vi "GetShapeResultNames.vi"(7 "ProjectName":string="Prj", 10 "SetParameter":T1={"Enum_ShapeType"=enum."Circles", "MaxParticle"=1, "Descriptor"={"Set 1"=100.0, "Set 2"=10.0, "Set 3"=200.0, "Set 4"=10.0}, "Match Options"={"Rotation"=TRUE, "Scale"=FALSE, "Occlusion"=FALSE, "Range Settings"=[{"Match Constraints"=0, "Min"=0.0, "Max"=360.0}]}, "Curve Parameters"={"Extraction Mode"=0, "Edge Threshold"=75, "Edge Filter Size"=1, "Min Length"=25, "Row Search Step Size"=15, "Col Search Step Size"=15, "Max Endpoint Gap"=10, "Closed"=FALSE, "Subpixel"=FALSE}, " score"=500.0} {"score" format="%#_15g"; "Curve Parameters"."Extraction Mode" items=["Normal", "Uniform Regions"]; "Curve Parameters"."Edge Filter Size" items=["Fine", "Normal"]; "Match Options"."Range Settings"."Match Constraints" items=["Rotation Angle (degrees)", "Scale Factor (%)", "Occlusion (%)"]}, 11 "ROI_Name":string="ROI1") -> (3 "ResultNames":string[](array[string]))   [LabVIEW 2019]
uses:
  Controls/Circle/Analysis_Circle_Result.ctl
  Controls/ShapeDectect/Analysis_ShapeDectect_Parameter.ctl
panel:
  in  "Tab Control":T2(tab)
  in  "Circles":T3
  in  "Ellipses":T4
  in  "Lines":T5
  in  "Rectangles":T6
  in  "Analysis_Clamp_Result":T7 {"Fitted Circle"."Average SNR (dB)" format="%.2f"; "Fitted Circle"."Average Strength" format="%.2f"; "Fitted Circle"."Roundness (Real-World)" format="%.2f"; "Fitted Circle"."Radius (Real-World)" format="%.2f"; "Fitted Circle"."Center (Real-World)"."Y" format="%.2f"; "Fitted Circle"."Center (Real-World)"."X" format="%.2f"; "Fitted Circle"."Radius (Pixels)" format="%.2f"; "Fitted Circle"."Center (Pixels)"."Y" format="%.2f"; "Fitted Circle"."Center (Pixels)"."X" format="%.2f"}
  out "error out":errorcluster
  in  "error in (no error)":errorcluster
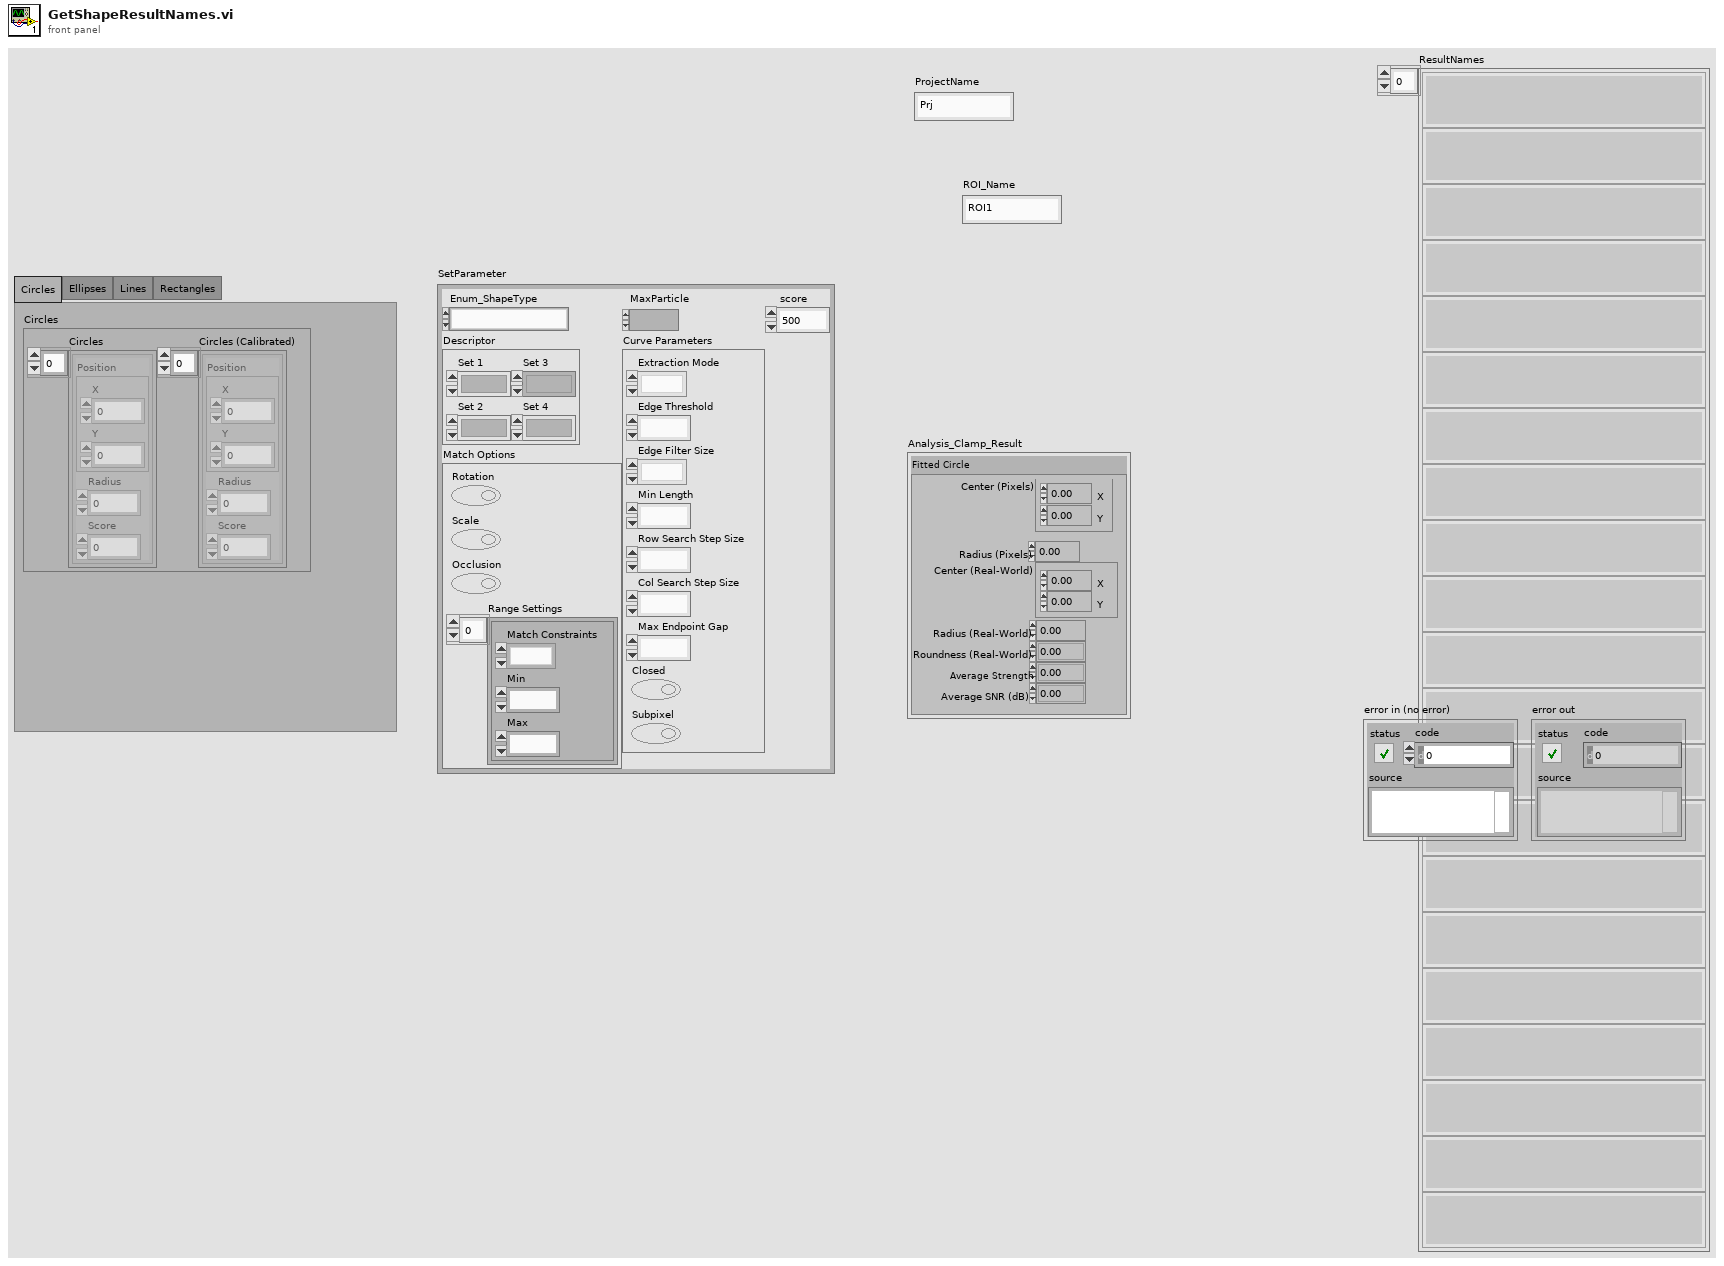
[diagram p1: front panel]
types:
  T1 = typedef "Analysis_ShapeDectect_Parameter.ctl" = cluster{"Enum_ShapeType":enum16{"Circles", "Ellipses", "Lines", "Rectangles"}, "MaxParticle":i32, "Descriptor":cluster{"Set 1":dbl, "Set 2":dbl, "Set 3":dbl, "Set 4":dbl}, "Match Options":cluster{"Rotation":bool, "Scale":bool, "Occlusion":bool, "Range Settings":cluster{"Match Constraints":u32, "Min":dbl, "Max":dbl}[]}, "Curve Parameters":cluster{"Extraction Mode":u32, "Edge Threshold":i32, "Edge Filter Size":u32, "Min Length":i32, "Row Search Step Size":i32, "Col Search Step Size":i32, "Max Endpoint Gap":i32, "Closed":bool, "Subpixel":bool}, " score":dbl}
  T2 = enum32{"Circles", "Ellipses", "Lines", "Rectangles"}
  T3 = cluster{"Circles":cluster{"Position":cluster{"X":sgl, "Y":sgl}, "Radius":dbl, "Score":dbl}[], "Circles (Calibrated)":cluster{"Position":cluster{"X":sgl, "Y":sgl}, "Radius":dbl, "Score":dbl}[]}
  T4 = cluster{"Pixel":cluster{"Position":cluster{"X":sgl, "Y":sgl}, "Angle":dbl, "Major Radius":dbl, "Minor Radius":dbl, "Score":dbl}[], "Ellipses (Calibrated)":cluster{"Position":cluster{"X":sgl, "Y":sgl}, "Orientation":dbl, "Major Radius":dbl, "Minor Radius":dbl, "Score":dbl}[]}
  T5 = cluster{"Lines":cluster{"Start Point":cluster{"X":sgl, "Y":sgl}, "End Point":cluster{"X":sgl, "Y":sgl}, "Length":dbl, "Angle":dbl, "Score":dbl}[], "Lines Calibrated":cluster{"Start Point":cluster{"X":sgl, "Y":sgl}, "End Point":cluster{"X":sgl, "Y":sgl}, "Length":dbl, "Orientation":dbl, "Score":dbl}[]}
  T6 = cluster{"Rectangles":cluster{"Corners":cluster{"X":sgl, "Y":sgl}[], "Angle":dbl, "Width":dbl, "Height":dbl, "Score":dbl}[], "Rectangles Calibrated":cluster{"Corners":cluster{"X":sgl, "Y":sgl}[], "Angle":dbl, "Width":dbl, "Height":dbl, "Score":dbl}[]}
  T7 = typedef "Analysis_Circle_Result.ctl" = cluster{"Fitted Circle":cluster{"Center (Pixels)":cluster{"X":sgl, "Y":sgl}, "Radius (Pixels)":dbl, "Center (Real-World)":cluster{"X":sgl, "Y":sgl}, "Radius (Real-World)":dbl, "Roundness (Real-World)":dbl, "Average Strength":dbl, "Average SNR (dB)":dbl}}
  T8 = enum16{"Circles", "Ellipses", "Lines", "Rectangles"}
  T9 = cluster{"Position":cluster{"X":sgl, "Y":sgl}, "Angle":dbl, "Major Radius":dbl, "Minor Radius":dbl, "Score":dbl}
  T10 = cluster{"Start Point":cluster{"X":sgl, "Y":sgl}, "End Point":cluster{"X":sgl, "Y":sgl}, "Length":dbl, "Angle":dbl, "Score":dbl}
  T11 = cluster{"Corners":cluster{"X":sgl, "Y":sgl}[], "Angle":dbl, "Width":dbl, "Height":dbl, "Score":dbl}
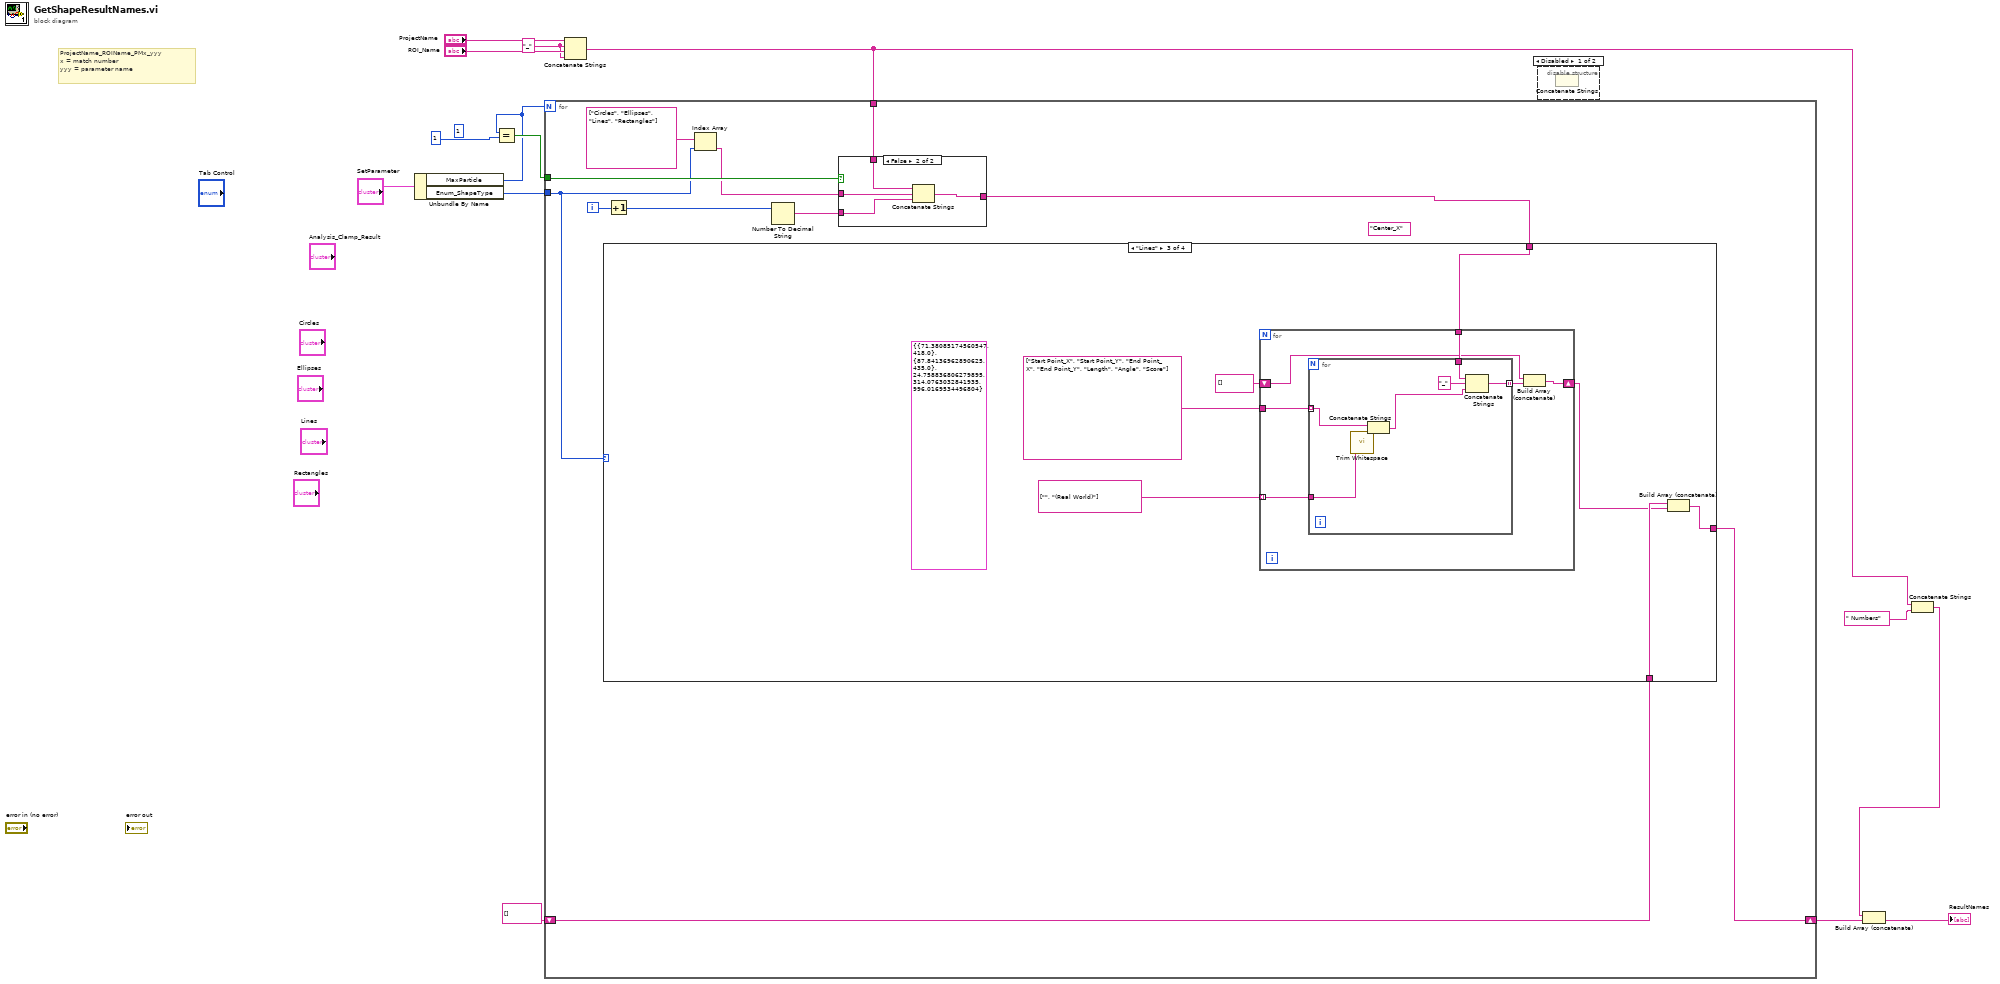
[diagram p0: block diagram]
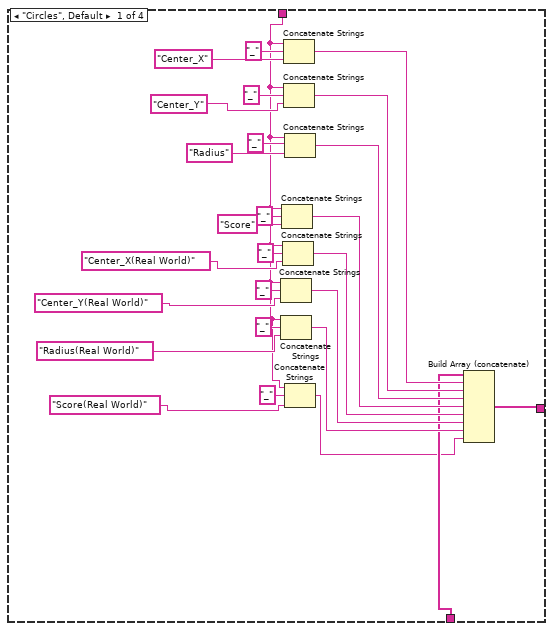
[diagram p3: hidden frame]
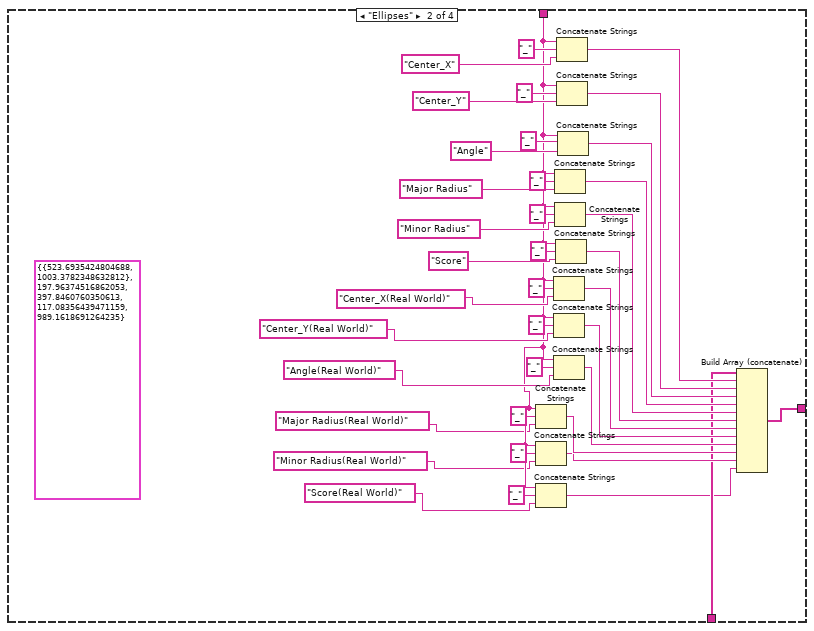
[diagram p4: hidden frame]
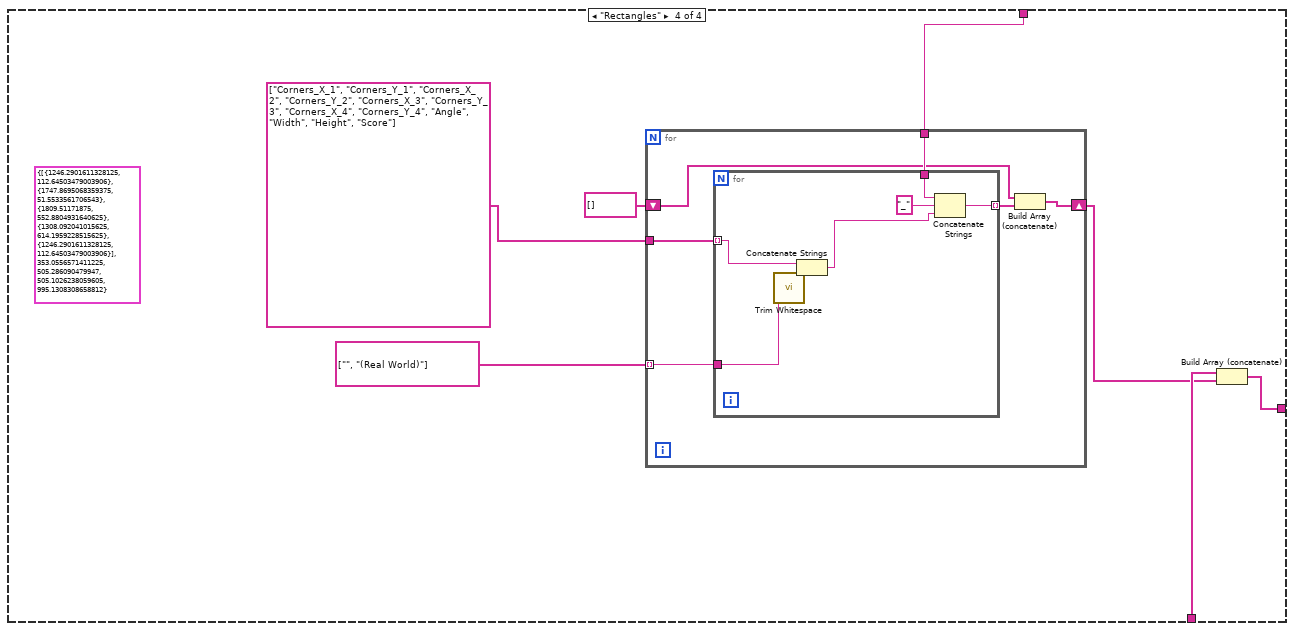
[diagram p5: hidden frame]
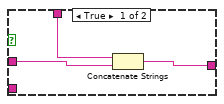
[diagram p6: hidden frame]
diagram:
  (unwired) 1 ("x")
  w12 = "_" ("string")
  # "ProjectName_ROIName_PMx_yyy\nx = match number\nyyy = parameter name"
  n1 = Unbundle By Name("SetParameter") -> ("MaxParticle"=w1:i32, "Enum_ShapeType"=w7:T8)
  n2 = Equal?(x=w1, y=1) -> (x = y?=w9:bool)
  n3 = Concatenate Strings("ProjectName", w12, "ROI_Name", w12) -> (w4:string)
  n4 = for {
    N: w1 -> [_]
    tunnel: w4 -> [w23]
    shift-right: [w19] -> w10
    shift-left: string[] [] -> [w20]
    tunnel: w9 -> [w24]
    tunnel: w7 -> [w15]
    i -> [w21]
    (unwired) "Center_X" ("string")
    n5 = Increment(x=w21) -> (x+1=w25:i32)
    n6 = Index Array(array=string[] ["Circles", "Ellipses", "Lines", "Rectangles"] ("Array"), index=w15) -> (element=w16:string)
    n7 = Number To Decimal String(number=w25) -> (decimal integer string=w22:string)  [unwired: 1 in]
    n8 = case shown="False" w24 {
      tunnel: w23 -> [w134 w138]
      tunnel: w22 -> [_ w136]
      tunnel: [w133 w137] -> w18
      tunnel: w16 -> [w132 w135]
      frame True {
        n9 = Concatenate Strings(w134, w132) -> (w133:string)
      }
      frame False {
        n10 = Concatenate Strings(w138, w135, w136) -> (w137:string)
      }
    }
    n11 = case shown="\"Lines\"" w15 {
      tunnel: w20 -> [w37 w54 w97 w117]
      tunnel: [w38 w91 w98 w118] -> w19
      tunnel: w18 -> [w28 w61 w94 w115]
      frame "Circles", Default {
        n12 = Concatenate Strings(w28, "_" ("string"), "Center_Y(Real World)" ("string")) -> (w48:string)
        n13 = Concatenate Strings(w28, "_" ("string"), "Radius(Real World)" ("string")) -> (w47:string)
        n14 = Concatenate Strings(w28, "_" ("string"), "Score" ("string")) -> (w50:string)
        n15 = Concatenate Strings(w28, "_" ("string"), "Center_X(Real World)" ("string")) -> (w49:string)
        n16 = Concatenate Strings(w28, "_" ("string"), "Center_X" ("string")) -> (w52:string)
        n17 = Concatenate Strings(w28, "_" ("string"), "Center_Y" ("string")) -> (w51:string)
        n18 = Concatenate Strings(w28, "_", "Radius" ("string")) -> (w39:string)
        n19 = Concatenate Strings(w28, "_" ("string"), "Score(Real World)" ("string")) -> (w26:string)
        n20 = Build Array (concatenate)(w37, w52, w51, w39, w50, w49, w48, w47, w26) -> (w38:string[])
      }
      frame "Ellipses" {
        (unwired) T9 {"Position"={"X"=523.69354, "Y"=1003.37823}, "Angle"=197.96374516862053, "Major Radius"=397.8460760350613, "Minor Radius"=117.08356439471159, "Score"=989.1618691264235} ("Circle Descriptor")
        n21 = Concatenate Strings(w61, "_" ("string"), "Major Radius(Real World)" ("string")) -> (w56:string)
        n22 = Concatenate Strings(w61, "_" ("string"), "Minor Radius(Real World)" ("string")) -> (w55:string)
        n23 = Concatenate Strings(w61, "_" ("string"), "Score(Real World)" ("string")) -> (w53:string)
        n24 = Concatenate Strings(w61, "_" ("string"), "Center_X(Real World)" ("string")) -> (w85:string)
        n25 = Concatenate Strings(w61, "_" ("string"), "Center_Y(Real World)" ("string")) -> (w84:string)
        n26 = Concatenate Strings(w61, "_" ("string"), "Angle(Real World)" ("string")) -> (w75:string)
        n27 = Concatenate Strings(w61, "_" ("string"), "Major Radius" ("string")) -> (w88:string)
        n28 = Concatenate Strings(w61, "_" ("string"), "Minor Radius" ("string")) -> (w87:string)
        n29 = Concatenate Strings(w61, "_" ("string"), "Score" ("string")) -> (w86:string)
        n30 = Concatenate Strings(w61, "_" ("string"), "Center_X" ("string")) -> (w90:string)
        n31 = Concatenate Strings(w61, "_" ("string"), "Center_Y" ("string")) -> (w89:string)
        n32 = Concatenate Strings(w61, "_", "Angle" ("string")) -> (w73:string)
        n33 = Build Array (concatenate)(w54, w90, w89, w73, w88, w87, w86, w85, w84, w75, w56, w55, w53) -> (w91:string[])
      }
      frame "Lines" {
        (unwired) T10 {"Start Point"={"X"=71.38085, "Y"=418.0}, "End Point"={"X"=87.84137, "Y"=435.0}, "Length"=24.758836806279895, "Angle"=314.0763032841935, "Score"=996.0169534496804} ("Circle Descriptor")
        n34 = for {
          tunnel: string[] ["Start Point_X", "Start Point_Y", "End Point_X", "End Point_Y", "Length", "Angle", "Score"] -> [w104]
          tunnel: string[] ["", "(Real World)"] -> [w103] mode=indexing
          tunnel: w94 -> [w102]
          shift-right: [w100] -> w92
          shift-left: string[] [] -> [w99]
          n35 = for {
            tunnel: w104 -> [w111] mode=indexing
            tunnel: w103 -> [w110]
            tunnel: w102 -> [w108]
            tunnel: [w105] -> w101 mode=indexing
            n36 = call <vilib>:"Trim Whitespace.vi"("string"=w110) -> ("trimmed string"=w106:string)  [unwired: 1 in]
            n37 = Concatenate Strings(w111, w106) -> (w107:string)
            n38 = Concatenate Strings(w108, "_" ("string"), w107) -> (w105:string)
          }
          n39 = Build Array (concatenate)(w99, w101) -> (w100:string[])
        }
        n40 = Build Array (concatenate)(w97, w92) -> (w98:string[])
      }
      frame "Rectangles" {
        (unwired) T11 {"Corners"=[{"X"=1246.2902, "Y"=112.645035}, {"X"=1747.8695, "Y"=51.553356}, {"X"=1809.5117, "Y"=552.8805}, {"X"=1308.092, "Y"=614.1959}, {"X"=1246.2902, "Y"=112.645035}], "Angle"=353.0556571411225, "Width"=505.286090479947, "Height"=505.1026238059605, "Score"=995.1308308658812} ("Rectangle Descriptor 2")
        n41 = for {
          tunnel: string[] ["Corners_X_1", "Corners_Y_1", "Corners_X_2", "Corners_Y_2", "Corners_X_3", "Corners_Y_3", "Corners_X_4", "Corners_Y_4", "Angle", "Width", "Height", "Score"] ("appended array") -> [w124]
          tunnel: string[] ["", "(Real World)"] -> [w123] mode=indexing
          tunnel: w115 -> [w122]
          shift-right: [w120] -> w113
          shift-left: string[] [] -> [w119]
          n42 = for {
            tunnel: w124 -> [w131] mode=indexing
            tunnel: w123 -> [w130]
            tunnel: w122 -> [w128]
            tunnel: [w125] -> w121 mode=indexing
            n43 = call <vilib>:"Trim Whitespace.vi"("string"=w130) -> ("trimmed string"=w126:string)  [unwired: 1 in]
            n44 = Concatenate Strings(w131, w126) -> (w127:string)
            n45 = Concatenate Strings(w128, "_" ("string"), w127) -> (w125:string)
          }
          n46 = Build Array (concatenate)(w119, w121) -> (w120:string[])
        }
        n47 = Build Array (concatenate)(w117, w113) -> (w118:string[])
      }
    }
  }
  n48 = disable-structure shown="Disabled" {
    frame Disabled {
      n49 = Concatenate Strings() -> ()  [unwired: 2 in, 1 out]
    }
    frame Enabled {
    }
  }
  n50 = Concatenate Strings(w4, " Numbers" ("string")) -> (w3:string)
  n51 = Build Array (concatenate)(w3, w10) -> (→"ResultNames":string[])
